vi "UHR-Fleezers Control (host) - 12.2.vi"() -> ()   [LabVIEW 2012] (continued)
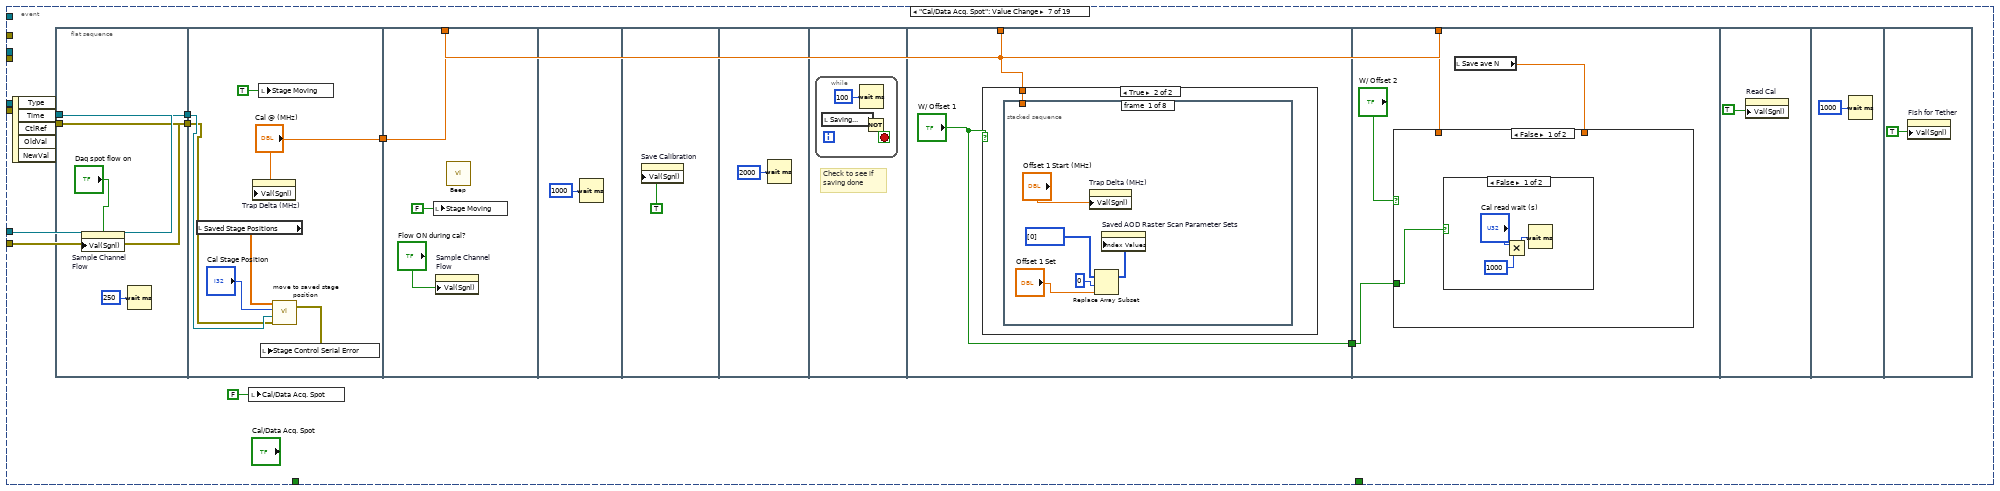
[diagram p15: hidden frame]
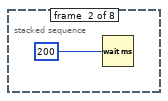
[diagram p17: hidden frame]
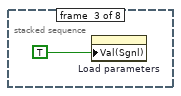
[diagram p18: hidden frame]
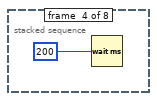
[diagram p19: hidden frame]
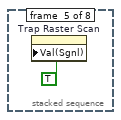
[diagram p20: hidden frame]
